vi "OnDone.vi"(8 "Error In":errorcluster, 11 "JSON Tree In":variant) -> (0 "Error Out":errorcluster, 3 "JSON Tree Out":variant)   [LabVIEW 2017, in "LiteAgentSDK.lvlib"]
uses:
  LiteAgentSDK.lvlib
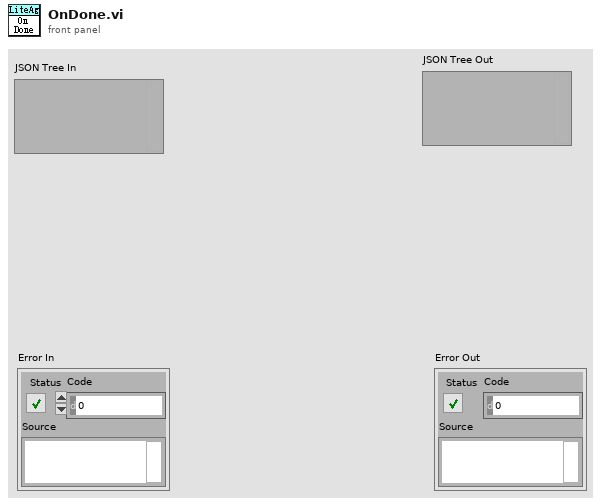
[diagram p1: front panel]
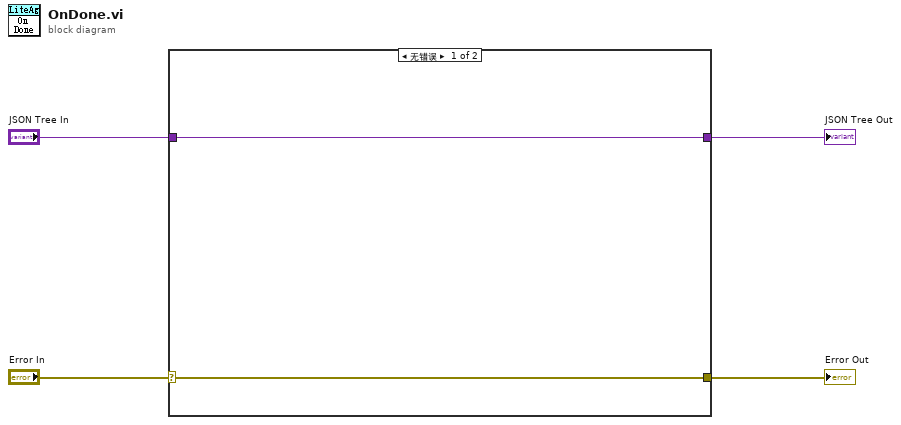
[diagram p0: block diagram]
diagram:
  n1 = case shown="无错误" "Error In" {
    selector: "Error In" -> [w5 w8]
    tunnel: [w5 w8] -> w3
    tunnel: "JSON Tree In" -> [w6 w7]
    tunnel: [w6 w7] -> w1
    frame No Error {
    }
    frame Error {
    }
  }
  "Error Out" <- w3
  "JSON Tree Out" <- w1
